vi "Write Sender.vi"(10 "Sender":refnum<class "Sender.lvclass">, 11 "Msg in":refnum<class "Msg.lvclass">) -> (3 "Msg out":refnum<class "Msg.lvclass">)   [LabVIEW 2020, in "jettl.lvlib" / "Msg.lvclass"]
uses:
  Msg.lvclass
  Sender/Sender/Sender.lvclass
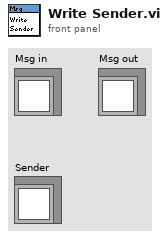
[diagram p1: front panel]
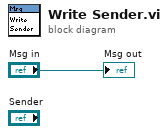
[diagram p0: block diagram]
diagram:
  "Msg out" <- "Msg in"
